vi "mbed-write.vi"(2 "Baud Rate":u32=9600, 3 "Serial Port":refnum<visa-resource-name>, 4 "Array of Numbers":dbl[](array[numeric]), 5 "Array of Strings":string[](array[string]), 6 "Number":dbl, 7 "Line String":string) -> (0 "Write Output":string)   [LabVIEW 2009]
uses:
  <vilib>/Instr/_visa.llb/VISA Set IO Buffer Mask.ctl
  <vilib>/Instr/_visa.llb/VISA Configure Serial Port (Instr).vi
panel:
  out "String from Array of Strings":string
  out "String From Array Of Numbers":string
  out "Number as String":string
  out "return count":u32
  out "Status":errorcluster
  out "VISA resource name out":refnum<visa-resource-name>
  # "mbed Write"
  # "http://mbed.org"
  # "Serial Settings"
  # "Input Data"
  # "Debug"
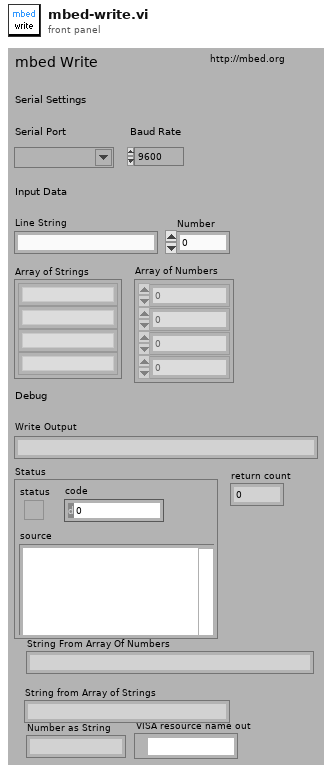
[diagram p1: front panel]
types:
  T1 = typedef "VISA Set IO Buffer Mask.ctl" = u16
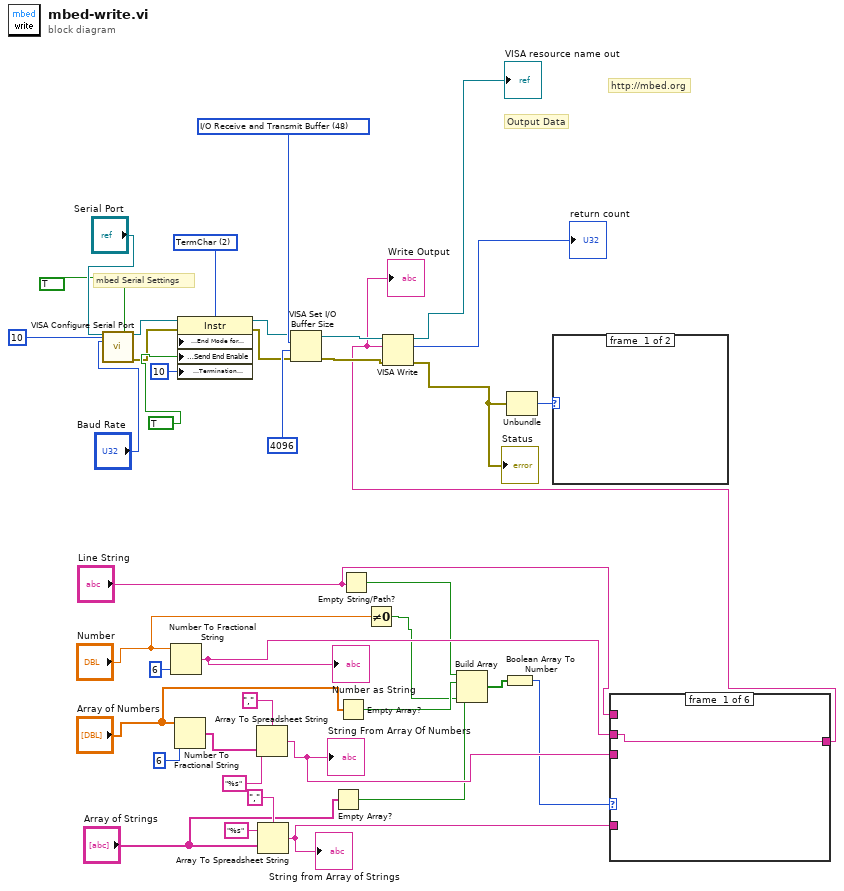
[diagram p0: block diagram]
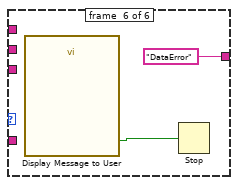
[diagram p6: hidden frame]
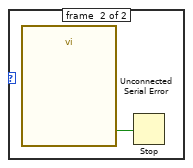
[diagram p7: hidden frame]
diagram:
  w31 = u16 2 items=["None", "Last Bit", "TermChar", "Break"] ("Serial Settings:End Mode for Writes")
  w35 = T1 48 items=["I/O Receive Buffer"=16, "I/O Transmit Buffer"=32, "I/O Receive and Transmit Buffer"=48] ("Mask")
  # "http://mbed.org"
  # "Output Data"
  # "mbed Serial Settings"
  n1 = call-poly "VISA Configure Serial Port"("VISA resource name"="Serial Port", "termination char\n(0xA = '\\n' = LF)"=u8 10 ("termination char\n(0xA = '\\n' = LF)"), "Enable Termination\nChar (T)"=TRUE ("Enable Termination\nChar (T)"), "baud rate (9600)"="Baud Rate") -> ("VISA resource name out"=w28:refnum<visa-resource-name>, "error out"=w26:errorcluster)  [unwired: 10 in]
  n2 = Number To Fractional String(number="Number", precision (6)=i16 6) -> (F-format string=w14:string)  [unwired: 2 in]
  "Number as String" <- w14
  n3 = Number To Fractional String(number="Array of Numbers", precision (6)=i16 6) -> (F-format string=w22:string[])  [unwired: 2 in]
  n4 = property class="Instr"(reference=w28, error in=w26, "Serial Settings:End Mode for Writes"=w31, "Message Based Settings:Send End Enable"=TRUE, "Message Based Settings:Termination Character"=u8 10) -> (reference out=w27:refnum<visa-resource-name>, error out=w25:errorcluster)
  n5 = Array To Spreadsheet String(delimiter (Tab)=",", array=w22, 3:"%s" ("format string")) -> (spreadsheet string=w12:string)
  "String From Array Of Numbers" <- w12
  n6 = Array To Spreadsheet String(delimiter (Tab)=",", array="Array of Strings", 3:"%s" ("format string")) -> (spreadsheet string=w13:string)
  "String from Array of Strings" <- w13
  n7 = VISA Set I/O Buffer Size(VISA resource name=w27, mask (16)=w35, size (4096)=u32 4096, error in (no error)=w25) -> (VISA resource name out=w37:refnum<visa-resource-name>, error out=w36:errorcluster)
  n8 = Empty Array?(array="Array of Strings") -> (empty?=w9:bool)
  n9 = Empty Array?(array="Array of Numbers") -> (empty?=w10:bool)
  n10 = Empty String/Path?(string/path="Line String") -> (empty?=w11:bool)
  n11 = Not Equal To 0?(x="Number") -> (x != 0?=w4:bool)
  n12 = Build Array(w11, w10, w9, w4) -> (w8:bool[])
  n13 = Boolean Array To Number(Boolean array=w8) -> (number=w7:u32)
  n14 = case shown="6" w7 {
    tunnel: "Line String" -> [_ _ w43 _ _ _]
    tunnel: w14 -> [w41 w42 _ _ _ _]
    tunnel: w12 -> [_ _ _ _ w45 _]
    tunnel: w13 -> [_ _ _ w44 _ _]
    tunnel: [w41 w42 w43 w44 w45 "DataError" ("spreadsheet string")] -> w6
    frame #0 {
    }
    frame #1 {
    }
    frame #2 {
    }
    frame #3 {
    }
    frame #4 {
    }
    frame #5 {
      n15 = call "Display Message to User"() -> ("OK"=w46:bool)  [unwired: 10 in, 1 out]
      n16 = Stop(stop? (T)=w46) -> ()
    }
  }
  "Write Output" <- w6
  n17 = VISA Write(VISA resource name=w37, write buffer=w6, error in (no error)=w36) -> (VISA resource name out=→"VISA resource name out":refnum<visa-resource-name>, return count=→"return count":u32, error out=w1:errorcluster)
  "Status" <- w1
  n18 = Unbundle(w1) -> ("code"=w39:i32)  [unwired: 2 out]
  n19 = case shown="1" w39 {
    frame #0 {
    }
    frame #1 {
      n20 = call "Unconnected Serial Error"() -> ("OK"=w48:bool)  [unwired: 10 in, 1 out]
      n21 = Stop(stop? (T)=w48) -> ()
    }
  }
